vi "solar Exit.vi"(8 "error in (no error)":errorcluster, 11 "solar in":refnum<class "solar.lvclass">) -> (0 "error out":errorcluster, 2 "Exit?":bool, 3 "solar out":refnum<class "solar.lvclass">)   [LabVIEW 2018, in "solar.lvclass"]
doc: "Handles the 'EXIT' command. <b>Exit?</b> must be set to true to shudown this target."
uses:
  solar.lvclass
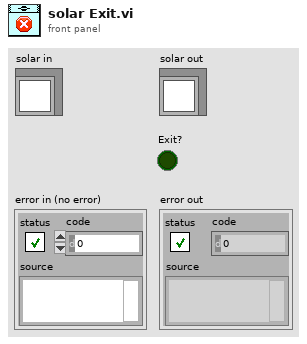
[diagram p1: front panel]
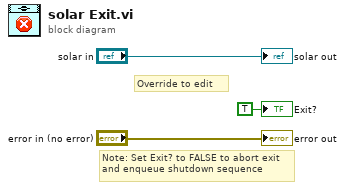
[diagram p0: block diagram]
diagram:
  # "Note: Set Exit? to FALSE to abort exit\nand enqueue shutdown sequence"
  # "Override to edit"
  "error out" <- "error in (no error)"
  "solar out" <- "solar in"
  "Exit?" <- TRUE ("Exit?")
